vi "N Channel N Samples - Auto Indexing.vi"() -> ()   [LabVIEW 2026, in "synnax_clib.lvlib"]
uses:
  lvlib/synnax_clib.lvlib
  lvlib/typedefs/connection_config.ctl
  lvlib/classes/Client/Private/synnax channel retrieve keys Array.vi
  lvlib/classes/Writer/Private/synnax writer open Array.vi
  lvlib/classes/Writer/Private/Writes/I32/Write NCh NSamp (I32).vi
  lvlib/classes/Synnax Writer.lvclass
  lvlib/classes/Client/Synnax Client.lvclass
panel:
  out "error out":errorcluster
  in  "Channels":string[](array[numeric])=["my_i32_ch1", "my_i32_ch2", "my_i32_ch3", "my_i32_ch4"]
  in  "Stop":bool
  in  "Connection Config":T1={"host"="localhost", "port"=9090, "username"="synnax", "password"="seldon"}
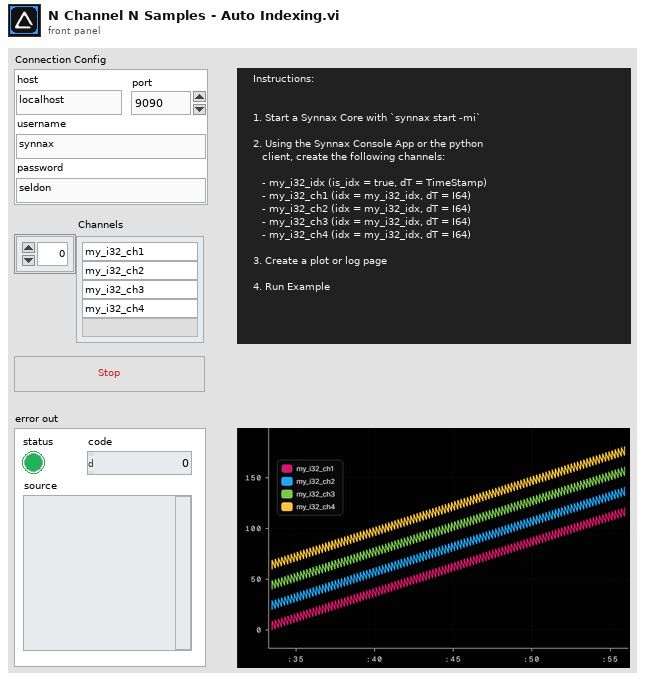
[diagram p1: front panel]
types:
  T1 = typedef "synnax_clib.lvlib/connection_config.ctl" = cluster{"host":string, "port":u16, "username":string, "password":string}
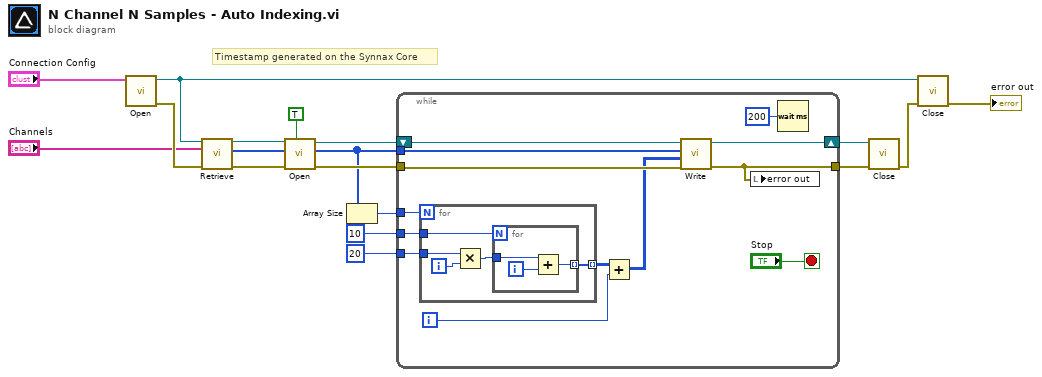
[diagram p0: block diagram]
diagram:
  # "Timestamp generated on the Synnax Core"
  n1 = call "Open.vi"("Connection Config"="Connection Config") -> ("error out"=w13:errorcluster, "Synnax Client out"=w15:refnum<class "Synnax Client.lvclass">)  [unwired: 9 in]
  n2 = call-poly "Retrieve.vi"("Synnax Client in"=w15, "channel names"="Channels", "error in"=w13) -> ("Synnax Client out"=w9:refnum<class "Synnax Client.lvclass">, "channel keys"=w8:u32[], "error out"=w17:errorcluster)  [unwired: 8 in, 2 out]
  n3 = call-poly "Open.vi"("auto_index (F)"=TRUE, "error in"=w17, "channels in"=w8, "Synnax Client in"=w9) -> ("error out"=w10:errorcluster, "channels out"=w6:u32[], "writer out"=w12:refnum<class "Synnax Writer.lvclass">)  [unwired: 5 in]
  n4 = Array Size(array=w6) -> (size(s)=w5:i32)
  n5 = while {
    shift-right: [w30] -> w11
    shift-left: w12 -> [w31]
    tunnel: w10 -> [w29]
    tunnel: [w26] -> w18
    tunnel: w6 -> [w24]
    tunnel: w5 -> [w23]
    tunnel: 10 -> [w22]
    tunnel: 20 -> [w19]
    i -> [w20]
    stop <- "Stop" stop-if-true
    n6 = for {
      N: w23 -> [_]
      tunnel: [w36] -> w27 mode=indexing
      tunnel: w22 -> [w32]
      tunnel: w19 -> [w33]
      i -> [w34]
      n7 = Multiply(x=w33, y=w34) -> (x*y=w35:i32)
      n8 = for {
        N: w32 -> [_]
        tunnel: [w37] -> w36 mode=indexing
        tunnel: w35 -> [w39]
        i -> [w38]
        n9 = Add(x=w39, y=w38) -> (x+y=w37:i32)
      }
    }
    n10 = Add(x=w27, y=w20) -> (x+y=w21:i32[][])
    n11 = call-poly "Write.vi"("error in"=w29, "data"=w21, "channels"=w24, "Writer"=w31) -> ("error out"=w26:errorcluster, "Writer Out"=w30:refnum<class "Synnax Writer.lvclass">)  [unwired: 6 in]
    n12 = local write "error out"(w26) -> ()
    n13 = Wait (ms)(milliseconds to wait=u32 200) -> ()  [unwired: 1 out]
  }
  n14 = call "Close.vi"("error in"=w18, "writer"=w11) -> ("error out"=w14:errorcluster)  [unwired: 9 in]
  n15 = call "Close.vi"("error in"=w14, "Synnax Client in"=w15) -> ("error out"=→"error out":errorcluster)  [unwired: 9 in]
